vi "horloge.vi"() -> ()   [LabVIEW 2025]
panel:
  out "SS":dbl(knob) scale=0.0..60.0
  out "MM":dbl(knob) scale=0.0..60.0
  out "HH":dbl(knob) scale=0.0..12.0
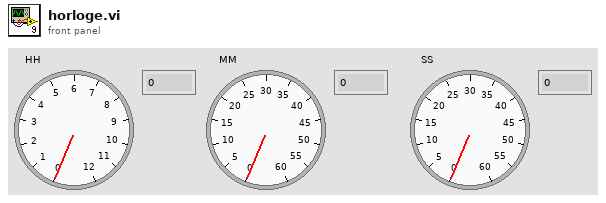
[diagram p1: front panel]
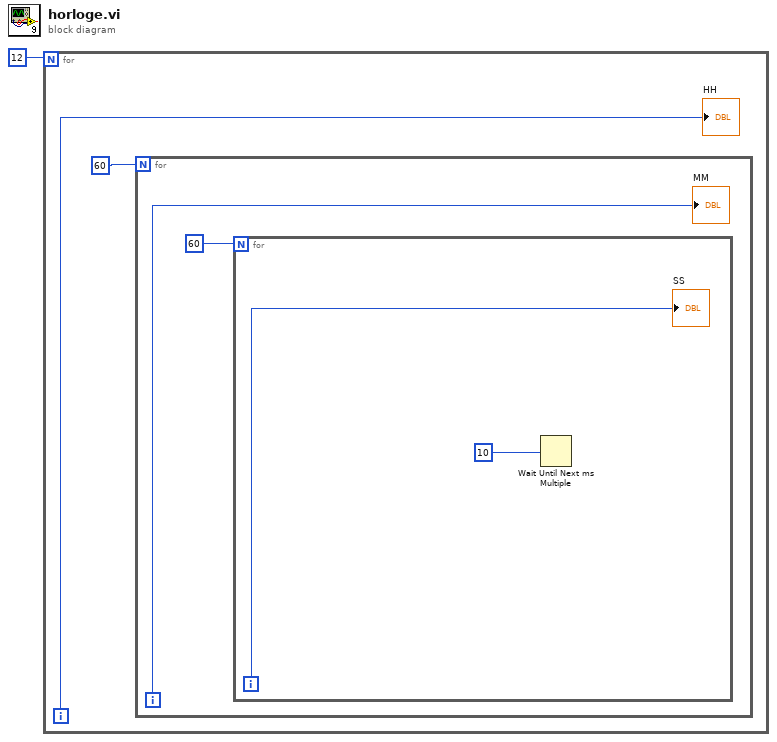
[diagram p0: block diagram]
diagram:
  n1 = for {
    N: 12 -> [_]
    i -> [w3]
    n2 = for {
      N: 60 -> [_]
      i -> [w5]
      n3 = for {
        N: 60 -> [_]
        i -> [w7]
        n4 = Wait Until Next ms Multiple(millisecond multiple=10) -> ()  [unwired: 1 out]
        "SS" <- w7
      }
      "MM" <- w5
    }
    "HH" <- w3
  }
